vi "Send command Get Pin.vi"(7 "Marca":string, 8 "error in (no error)":errorcluster, 9 "Pin":string, 10 "Puerto":string, 11 "NXP in":refnum<class "NXP.lvclass">) -> (0 "error out":errorcluster, 1 "Command":string, 2 "Expected response":string, 3 "NXP out":refnum<class "NXP.lvclass">)   [LabVIEW 2020, in "NXP.lvclass"]
doc: "Se manda el comando para leer obtener el status del pin, se escribe en el puerto serial y se lee la respuesta que de el micro."
uses:
  NXP.lvclass
  D:/Fork/IVProyecto_3P/Abstract/Serial Device/Serial Device.lvclass
  NXP.lvclass/NXP.ctl
  Abstract/Serial Device/Serial Device.lvclass
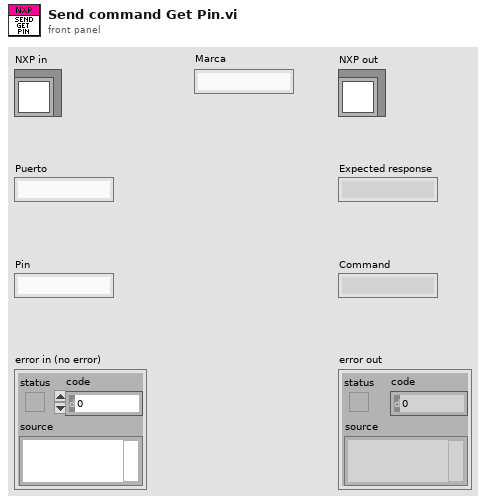
[diagram p1: front panel]
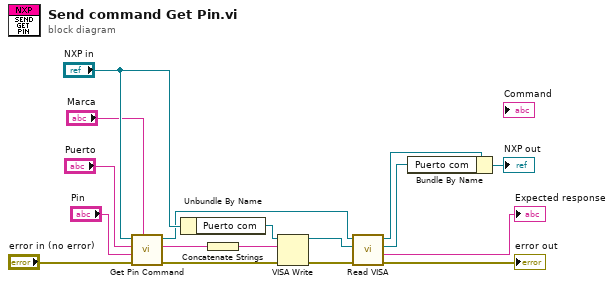
[diagram p0: block diagram]
diagram:
  n1 = call "Get Pin Command.vi"("Marca"="Marca", "error in (no error)"="error in (no error)", "Pin"="Pin", "Puerto"="Puerto", "Serial Device in"="NXP in") -> ("error out"=w5:errorcluster, "Command"=w6:string, "Serial Device out"=w7:refnum<class "NXP.lvclass">)  [unwired: 3 in, 1 out]
  n2 = Unbundle By Name("NXP in") -> ("Puerto com"=w15:refnum<visa-resource-name>)
  n3 = Concatenate Strings(w6) -> (w16:string)
  n4 = VISA Write(VISA resource name=w15, write buffer=w16, error in (no error)=w5) -> (VISA resource name out=w14:refnum<visa-resource-name>, error out=w17:errorcluster)  [unwired: 1 out]
  n5 = call-dynamic "Read VISA.vi"("error in (no error)"=w17, "VISA Refnum in"=w14, "Serial Device in"=w7) -> ("error out"=→"error out":errorcluster, "Serial Response"=→"Expected response":string, "VISA resource name out"=w12:refnum<visa-resource-name>, "Serial Device out"=w13:refnum<class "NXP.lvclass">)  [unwired: 5 in]
  n6 = Bundle By Name(cluster=w13, "Puerto com"=w12) -> (→"NXP out":refnum<class "NXP.lvclass">)
